vi "MarvinReport.vi"(0 "HEADER1":string="===================================================================\r\n||  Functional and Performance Test  For  DUAL-SERVO- L O W E R  ||\r\n||  P/N  TLM132XX501    S/N:001    Power-Input:18,28,32 +/-0.5V  ||\r\n||  Date:6/12/2007    Time: 15-00  Test-Conductor: Itzik         ||\r\n||  Tester P/N yyyy-yyyyyy-yyyy    S/N:01                        ||\r\n||  POWER SUPPLY P/N xxxxx                                       ||\r\n||  Remarks:                                                     ||\r\n||  You can write here what ever you want                        ||\r\n||                                                               ||\r\n===================================================================", 1 "ATR Or":refnum<vi>, 2 "Steps   pfull":string[][](table)=array602x15[9030 elements] caption="ATR", 5 "pageNum":i32=13, 7 "FILE NAME":string="d", 9 "Report Folder":path=path "C:/EPD/ATRS", 11 "Open File":bool caption="Open", 12 "error in (no error)":errorcluster, 14 "Test-Conductor":string) -> (4 "path out":path, 15 "error out":errorcluster)   [LabVIEW 2017]
uses:
  <vilib>/Utility/miscctls.llb/LVRowAndColumnUnsignedTypeDef.ctl
  <vilib>/Utility/NIReport.llb/Append Report Text (str wrap).vi
  <vilib>/Utility/NIReport.llb/NI_report.lvclass
  <vilib>/Utility/NIReport.llb/Word/NI_Word.lvclass
panel:
  out "error out 2":errorcluster
  out "RefArr":u32[](array[numeric])
  in  "Tab Control":T1(tab)=enum."Headers and more"
  out "ERRORS\nLIST":string="<pre>Summery of Results (Fails Only) :   Pos.Cmnd.=0.5V F.B. - FAIL !\t   \nPos.Cmnd.=2.0V F.B. - FAIL !\t       Pos.Cmnd.=4.5V F.B. - FAIL !\t  \nPos.Cmnd.=0.5V F.B  - FAIL !\t       Pos.Cmnd.=2.0V F.B. - FAIL !\t\nPos.Cmnd.=4.5V F.B. - FAIL !\t       Pot. / Pos.Cmnd. 1.5v - FAIL !\t   \nPot./Pos.Cmnd.2.0v  - FAIL !\t       Pot. / Pos.Cmnd. 3.5v - FAIL !\t   \nRelay-->RESET  - FAIL !\t            Relay --> SET - FAIL !\t</pre>"
  out "Steps   p1":string[][](table)=[["Load Firmware - reset", "-", "-", "-", "-", ""], ["Test Communication", "-", "-", "-", "-", ""], ["Set S/N", "-", "-", "-", "-", ""], ["Set Board Number", "-", "-", "-", "-", ""], [" ", "", "", "", "", ""], ["Test Communication", "-", "-", "-", "-", ""], ["Get S/N", "-", "-", "-", "", ""], ["Get Board Number", "-", "-", "-", "", ""], ["Get FW", "-", "-", "-", "", ""], ["Small position command", "", "", "", "", ""], ["Measure delta", "", "", "", "", ""], ["Velocity command", "", "", "", "", ""], ["Velocity command", "", "", "", "", ""], ["Velocity command", "", "", "", "", ""], ["Velocity command", "", "", "", "", ""], ["Velocity command", "", "", "", "", ""]] caption="ATR"
  out "Steps   p2":string[][](table)=[["Load Firmware - reset", "-", "-", "-", "-", ""], ["Test Communication", "-", "-", "-", "-", ""], ["Set S/N", "-", "-", "-", "-", ""], ["Set Board Number", "-", "-", "-", "-", ""], [" ", "", "", "", "", ""], ["Test Communication", "-", "-", "-", "-", ""], ["Get S/N", "-", "-", "-", "", ""], ["Get Board Number", "-", "-", "-", "", ""], ["Get FW", "-", "-", "-", "", ""], ["Small position command", "", "", "", "", ""], ["Measure delta", "", "", "", "", ""], ["Velocity command", "", "", "", "", ""], ["Velocity command", "", "", "", "", ""], ["Velocity command", "", "", "", "", ""], ["Velocity command", "", "", "", "", ""], ["Velocity command", "", "", "", "", ""]] caption="ATR"
  out "Steps   p3":string[][](table) caption="ATR"
  in  "Fail  Button":bool
  in  "Pass  Button":bool
  # "e"
  # "e"
  # "<pre>"
  # "for html"
  # "for html"
  # "</pre>"
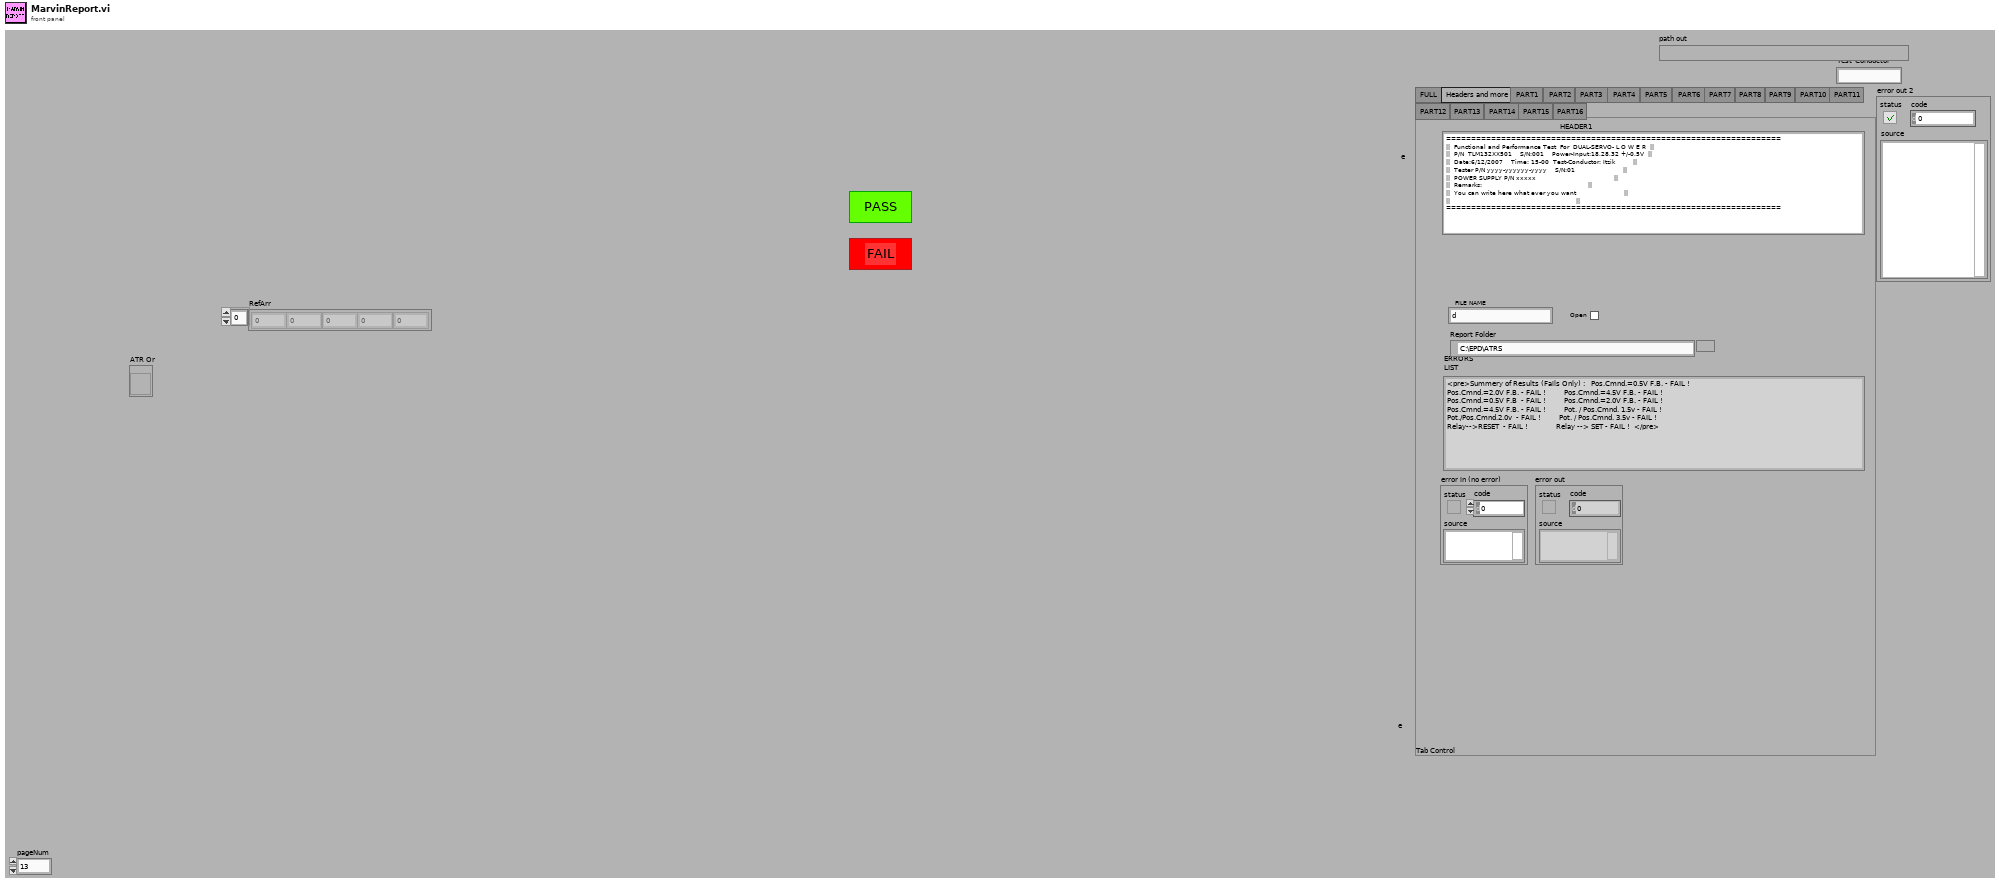
[diagram p1: front panel]
types:
  T1 = enum32{"FULL", "Headers and more", "PART1 ", "PART2 ", "PART3 ", "PART4 ", "PART5 ", "PART6 ", "PART7", "PART8", "PART9", "PART10", "PART11", "PART12", "PART13", "PART14", "PART15", "PART16"}
  T2 = typedef "LVRowAndColumnUnsignedTypeDef.ctl" = cluster{"Row":u32, "Column":u32}
  T3 = enum16{"Standard Report", "HTML", "Word", "Excel"}
  T4 = cluster{"Italic":enum16{"Italic Unchanged", "Italic On", "Italic Off"}, "Strike Through":enum16{"Strike Through Unchanged", "Strike Through On", "Strike Through Off"}, "Underline":enum16{"Underline Unchanged", "Underline On", "Underline Off"}, "Bold":enum16{"Bold Unchanged", "Bold On", "Bold Off"}}
  T5 = cluster{"charset (-1)":i16, "weight (-1)":i16, "name":string, "size":string}
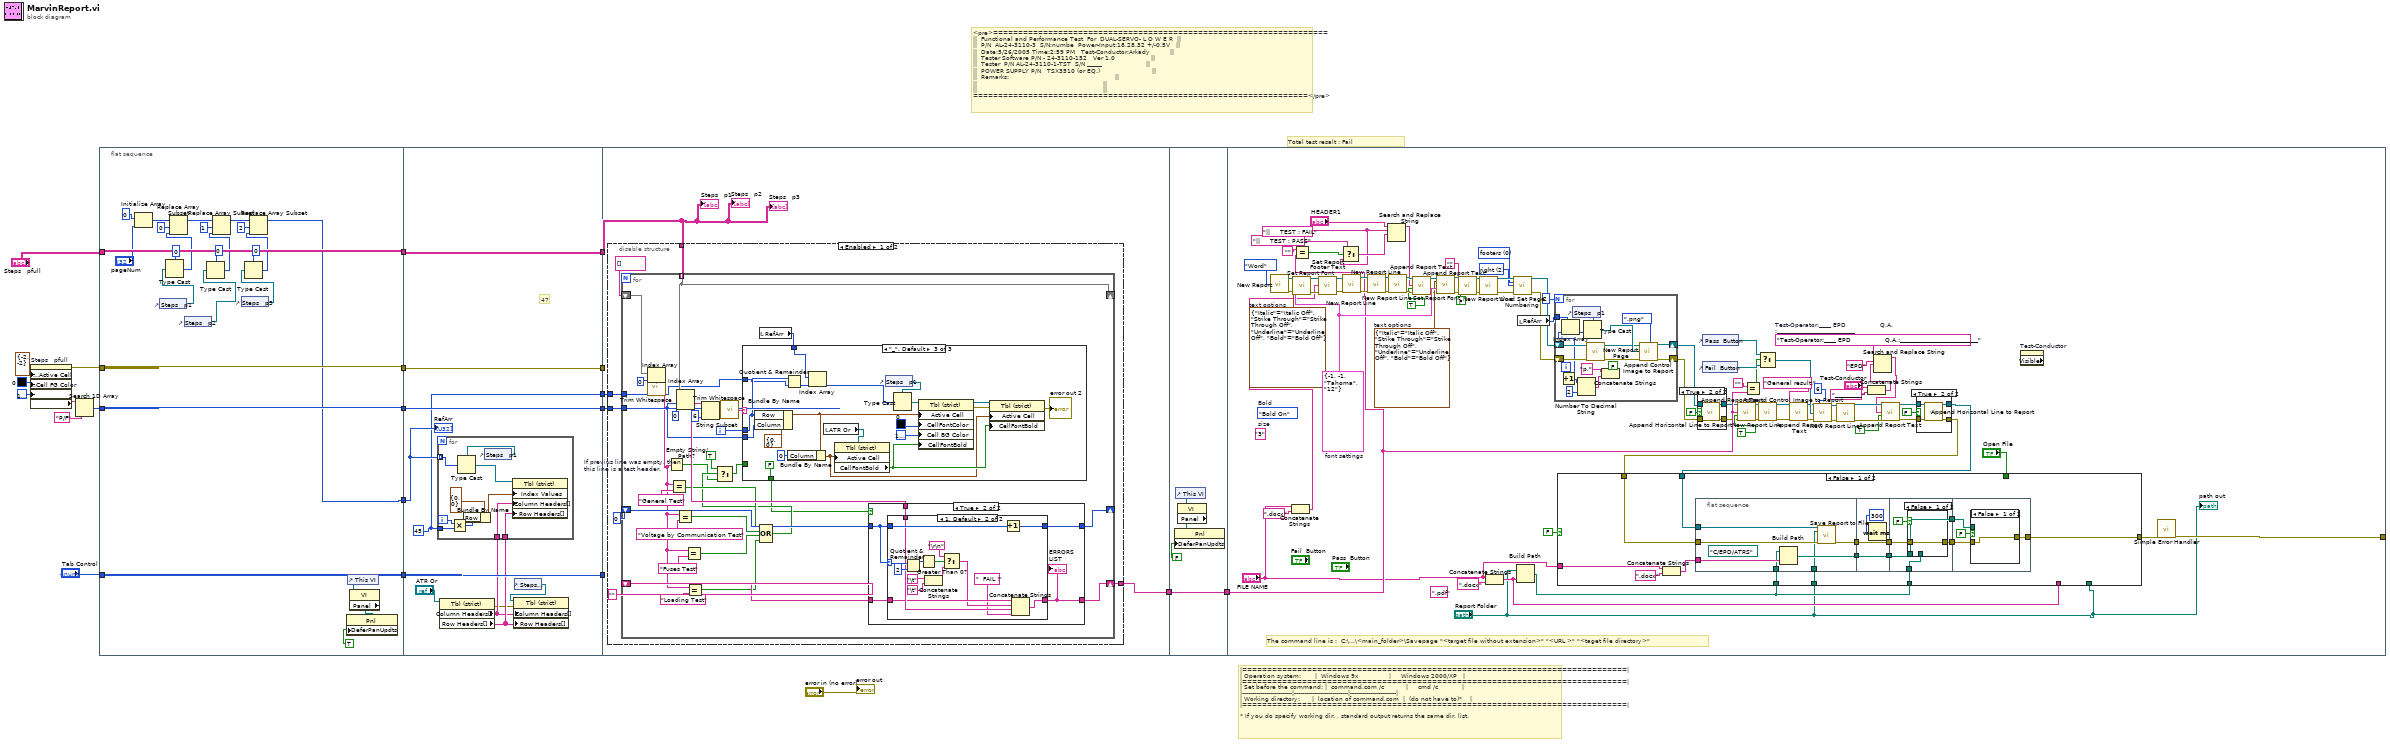
[diagram p0: block diagram]
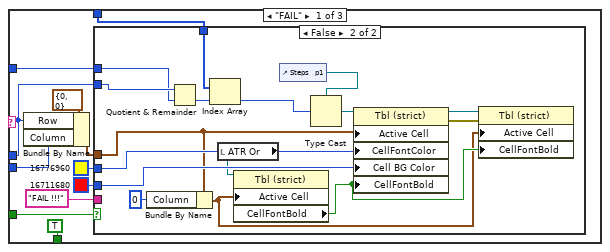
[diagram p2: hidden frame]
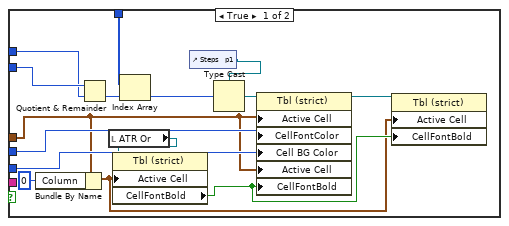
[diagram p3: hidden frame]
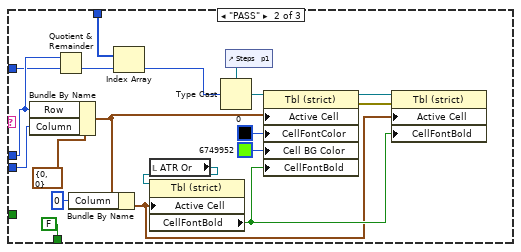
[diagram p4: hidden frame]
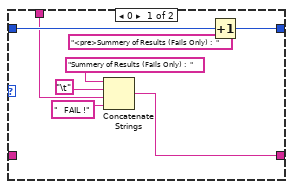
[diagram p6: hidden frame]
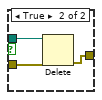
[diagram p9: hidden frame]
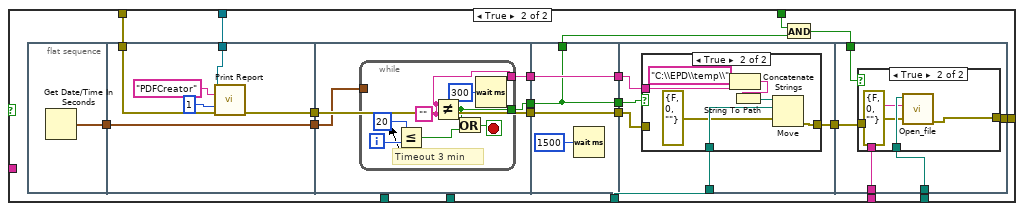
[diagram p10: hidden frame]
diagram:
  # "Total test resalt : Fail"
  # "|=============================================================================|\n| Operation system:       |  Windows 9x               |     Windows 2000/XP   |\n|=============================================================================|\n| Set before the command: |  command.com /c           |     cmd /c            |\n|-------------------------|---------------------------|-----------------------|\n| Working directory:      |  location of command.com  |  (do not have to)*    |\n|=============================================================================|\n\n* If you do specify working dir. , standard output returns the same dir. list."
  # "<pre>===================================================================\n||  Functional and Performance Test  For  DUAL-SERVO- L O W E R  ||\n||  P/N  AL-24-3110-3  S/N:numbe  Power-Input:18,28,32 +/-0.5V   ||\n||  Date:5/26/2005 Time:2:59 PM   Test-Conductor:Arkady          ||\n||  Tester Software P/N - 24-3110-152   Ver 1.0                  ||\n||  Tester  P/N AL-24-3110-1-TST  S/N _____                      ||\n||  POWER SUPPLY P/N   TSX3510 (or EQ.)                          ||\n||  Remarks:                                                     ||\n||                                                               ||\n||                                                               ||\n===================================================================</pre>"
  n1 = property on="Steps   pfull" class="Tbl (strict)"("Active Cell:Active Cell"=cluster{"Row":i32, "Column":i32} {"Row"=-2, "Column"=-2} ("Active Cell"), "Active Cell:Cell FG Color"=u32 0, "Active Cell:Cell Background Color"=u32 16777226) -> (error out=w19:errorcluster, "Column Header Strings[]"=w17:string[])  [unwired: 2 in, 1 out]
  n2 = Search 1D Array(1D array=w17, element="P/F") -> (index of element=w16:i32)  [unwired: 1 in]
  n3 = flat-sequence {
    tunnel: "Tab Control" -> [w44]
    tunnel: w16 -> [w45]
    tunnel: w19 -> [w46]
    tunnel: "Steps   pfull" -> [w47]
    tunnel: [w47] -> w8
    tunnel: [w46] -> w7
    tunnel: [w45] -> w6
    tunnel: [w44] -> w5
    tunnel: [w23] -> w2
    tunnel: [w58] -> w12
    tunnel: [w57] -> w11
    tunnel: [w56] -> w10
    tunnel: [w55] -> w9
    tunnel: w8 -> [w58]
    tunnel: w7 -> [w57]
    tunnel: w6 -> [w56]
    tunnel: w5 -> [w55]
    tunnel: w2 -> [w50]
    tunnel: [w48] -> w1
    tunnel: [w71] -> w4
    tunnel: w12 -> [w70]
    tunnel: w11 -> [_]
    tunnel: w10 -> [w72]
    tunnel: w9 -> [_]
    tunnel: w1 -> [w69]
    tunnel: w4 -> [w225]
    tunnel: [w225] -> w3
    tunnel: [w309] -> _
    tunnel: w3 -> [w271]
    frame #0 {
      n4 = Initialize Array "Initialize Array"(u32 0, "pageNum") -> (w28:u32[])
      n5 = control-ref of="Steps   p1"() -> (w40:refnum<vi>)
      n6 = Type Cast(type=u32 0, x=w40) -> (*(type *) &x=w29:u32)
      n7 = Replace Array Subset(array=w28, new element=w29, index=0) -> (w32:u32[])
      n8 = control-ref of="Steps   p2"() -> (w24:refnum<vi>)
      n9 = Type Cast(type=u32 0, x=w24) -> (*(type *) &x=w33:u32)
      n10 = Replace Array Subset(array=w32, new element=w33, index=1) -> (w38:u32[])
      n11 = control-ref of="Steps   p3"() -> (w39:refnum<vi>)
      n12 = Type Cast(type=u32 0, x=w39) -> (*(type *) &x=w36:u32)
      n13 = Replace Array Subset(array=w38, new element=w36, index=2) -> (w23:u32[])
      n14 = control-ref of="This VI"() -> (w41:refnum<vi>)
      n15 = property class="VI"(reference=w41) -> ("Panel"=w42:refnum<vi>)  [unwired: 1 in, 2 out]
      n16 = property class="Pnl"(reference=w42, "DeferPanUpdts"=TRUE ("Defer Panel Updates")) -> ()  [unwired: 1 in, 2 out]
    }
    frame #1 {
      w48 = u32 45 ("Row")
      # "47"
      n17 = property class="Tbl (strict)"(reference="ATR Or") -> (error out=w52:errorcluster, "Column Headers[]"=w53:string[], "Row Headers[]"=w54:string[])  [unwired: 1 in, 1 out]
      n18 = for {
        tunnel: w50 -> [w68] mode=indexing
        tunnel: w53 -> [w62]
        tunnel: w54 -> [w61]
        tunnel: w48 -> [w59]
        i -> [w64]
        n19 = Multiply(x=w64, y=w59) -> (x*y=w63:u32)
        n20 = Bundle By Name(cluster=T2 {"Row"=0, "Column"=0} ("Index Values"), "Row"=w63) -> (w65:T2)
        n21 = control-ref of="Steps   p1"() -> (w60:refnum<vi>)
        n22 = Type Cast(type=w60, x=w68) -> (*(type *) &x=w67:refnum<vi>)
        n23 = property class="Tbl (strict)"(reference=w67, "Index Values"=w65, "Column Headers[]"=w62, "Row Headers[]"=w61) -> ()  [unwired: 1 in, 2 out]
      }
      n24 = control-ref of="Steps   pfull"() -> (w49:refnum<vi>)
      n25 = property class="Tbl (strict)"(reference=w49, error in=w52, "Column Headers[]"=w53, "Row Headers[]"=w54) -> ()  [unwired: 2 out]
      "RefArr" <- w50
    }
    frame #2 {
      n26 = disable-structure shown="Enabled" {
        disable-tunnel: w72 -> [w79 _]
        disable-tunnel: [w78 _] -> w71
        disable-tunnel: w70 -> [w74 _]
        disable-tunnel: w69 -> [w73 _]
        frame Enabled {
          n27 = for {
            tunnel: w74 -> [w109] mode=indexing
            shift-right: [w109] -> _
            shift-left: string[] [] ("ATR in") -> [w108]
            tunnel: w79 -> [w85]
            shift-right: [w100] -> w78
            shift-left: "" ("trimmed string") -> [w104]
            shift-right: [w103] -> _
            shift-left: 0 -> [w102]
            tunnel: w73 -> [w80]
            i -> [w86]
            n28 = Index Array(array=w108, index=0) -> (element=w106:string)
            n29 = call <vilib>:"Trim Whitespace.vi"("string"=w106) -> ("trimmed string"=w81:string)  [unwired: 1 in]
            n30 = Empty String/Path? "If previus line was empty, then\nthis line is a test header."(string/path=w81) -> (empty?=w88:bool)
            n31 = Equal?(x=w81, y="General Test") -> (x = y?=w97:bool)
            n32 = Equal?(x=w81, y="Voltage by Communication Test") -> (x = y?=w92:bool)
            n33 = Index Array(array=w109, index #1=w85, index #2=0) -> (element #1=w105:string, element #2=w101:string)
            n34 = Equal?(x=w81, y="Fuses Test") -> (x = y?=w93:bool)
            n35 = Equal?(x=w81, y="Loading Test") -> (x = y?=w94:bool)
            n36 = String Subset(string=w105, length (rest)=6 ("length (rest)")) -> (substring=w110:string)  [unwired: 1 in]
            n37 = call <vilib>:"Trim Whitespace.vi"("string"=w110) -> ("trimmed string"=w87:string)  [unwired: 1 in]
            n38 = local read "RefArr"() -> (w82:u32[])
            n39 = Compound Arithmetic op=OR(w97, w92, w93, w94) -> (w95:bool)
            n40 = Select(t=TRUE, s=w95, f=w88) -> (s? t:f=w84:bool)
            n41 = case shown="\"_\", Default" w87 {
              tunnel: w86 -> [w114 w167 w188]
              tunnel: w85 -> [w116 w171 w191]
              tunnel: w84 -> [w118 _ _]
              tunnel: [TRUE FALSE FALSE] -> w83
              tunnel: w82 -> [w115 w165 w187]
              tunnel: w80 -> [w112 w154 w173]
              frame "FAIL" {
                n42 = Bundle By Name(cluster=cluster{"Row":i32, "Column":i32} {"Row"=0, "Column"=0} ("Active Cell"), "Row"=w114, "Column"=w116) -> (w122:cluster{"Row":i32, "Column":i32})
                n43 = case shown="False" w118 {
                  tunnel: w122 -> [w130 w142]
                  tunnel: u32 16776960 -> [w137 w153]
                  tunnel: u32 16711680 -> [w136 w152]
                  tunnel: "FAIL !!!" ("string") -> [_ _]
                  tunnel: w115 -> [w134 w149]
                  tunnel: w114 -> [w133 w150]
                  tunnel: w112 -> [w123 w138]
                  frame True {
                    n44 = Bundle By Name(cluster=w130, "Column"=0) -> (w126:cluster{"Row":i32, "Column":i32})
                    n45 = Quotient & Remainder(x=w133, y=w123) -> (floor(x/y)=w135:u32)  [unwired: 1 out]
                    n46 = local read "ATR Or"() -> (w124:refnum<vi>)
                    n47 = property class="Tbl (strict)"(reference=w124, "Active Cell"=w126) -> ("CellFontBold"=w127:bool)  [unwired: 1 in, 2 out]
                    n48 = Index Array(array=w134, index=w135) -> (element=w131:u32)
                    n49 = control-ref of="Steps   p1"() -> (w125:refnum<vi>)
                    n50 = Type Cast(type=w125, x=w131) -> (*(type *) &x=w132:refnum<vi>)
                    n51 = property class="Tbl (strict)"(reference=w132, "Active Cell"=w130, "CellFontColor"=w137, "Cell BG Color"=w136, "Active Cell"=w130, "CellFontBold"=w127) -> (reference out=w128:refnum<vi>)  [unwired: 1 in, 1 out]
                    n52 = property class="Tbl (strict)"(reference=w128, "Active Cell"=w126, "CellFontBold"=w127) -> ()  [unwired: 1 in, 2 out]
                  }
                  frame False {
                    n53 = Bundle By Name(cluster=w142, "Column"=0) -> (w141:cluster{"Row":i32, "Column":i32})
                    n54 = Quotient & Remainder(x=w150, y=w138) -> (floor(x/y)=w151:u32)  [unwired: 1 out]
                    n55 = Index Array(array=w149, index=w151) -> (element=w148:u32)
                    n56 = local read "ATR Or"() -> (w140:refnum<vi>)
                    n57 = property class="Tbl (strict)"(reference=w140, "Active Cell"=w141) -> ("CellFontBold"=w144:bool)  [unwired: 1 in, 2 out]
                    n58 = control-ref of="Steps   p1"() -> (w139:refnum<vi>)
                    n59 = Type Cast(type=w139, x=w148) -> (*(type *) &x=w147:refnum<vi>)
                    n60 = property class="Tbl (strict)"(reference=w147, "Active Cell"=w142, "CellFontColor"=w153, "Cell BG Color"=w152, "CellFontBold"=w144) -> (reference out=w146:refnum<vi>, error out=w145:errorcluster)  [unwired: 1 in]
                    n61 = property class="Tbl (strict)"(reference=w146, error in=w145, "Active Cell"=w141, "CellFontBold"=w144) -> ()  [unwired: 2 out]
                  }
                }
              }
              frame "PASS" {
                n62 = Bundle By Name(cluster=cluster{"Row":i32, "Column":i32} {"Row"=0, "Column"=0} ("Active Cell"), "Row"=w167, "Column"=w171) -> (w158:cluster{"Row":i32, "Column":i32})
                n63 = Quotient & Remainder(x=w167, y=w154) -> (floor(x/y)=w166:u32)  [unwired: 1 out]
                n64 = Bundle By Name(cluster=w158, "Column"=0) -> (w157:cluster{"Row":i32, "Column":i32})
                n65 = Index Array(array=w165, index=w166) -> (element=w164:u32)
                n66 = local read "ATR Or"() -> (w155:refnum<vi>)
                n67 = property class="Tbl (strict)"(reference=w155, "Active Cell"=w157) -> ("CellFontBold"=w160:bool)  [unwired: 1 in, 2 out]
                n68 = control-ref of="Steps   p1"() -> (w156:refnum<vi>)
                n69 = Type Cast(type=w156, x=w164) -> (*(type *) &x=w163:refnum<vi>)
                n70 = property class="Tbl (strict)"(reference=w163, "Active Cell"=w158, "CellFontColor"=u32 0, "Cell BG Color"=u32 6749952, "CellFontBold"=w160) -> (reference out=w161:refnum<vi>, error out=w162:errorcluster)  [unwired: 1 in]
                n71 = property class="Tbl (strict)"(reference=w161, error in=w162, "Active Cell"=w157, "CellFontBold"=w160) -> ()  [unwired: 2 out]
              }
              frame "_", Default {
                n72 = Bundle By Name(cluster=cluster{"Row":i32, "Column":i32} {"Row"=0, "Column"=0} ("Active Cell"), "Row"=w188, "Column"=w191) -> (w181:cluster{"Row":i32, "Column":i32})
                n73 = Quotient & Remainder(x=w188, y=w173) -> (floor(x/y)=w189:u32)  [unwired: 1 out]
                n74 = Bundle By Name(cluster=w181, "Column"=0) -> (w177:cluster{"Row":i32, "Column":i32})
                n75 = Index Array(array=w187, index=w189) -> (element=w186:u32)
                n76 = local read "ATR Or"() -> (w175:refnum<vi>)
                n77 = property class="Tbl (strict)"(reference=w175, "Active Cell"=w177) -> ("CellFontBold"=w178:bool)  [unwired: 1 in, 2 out]
                n78 = control-ref of="Steps   p1"() -> (w176:refnum<vi>)
                n79 = Type Cast(type=w176, x=w186) -> (*(type *) &x=w183:refnum<vi>)
                n80 = property class="Tbl (strict)"(reference=w183, "Active Cell"=w181, "CellFontColor"=u32 0, "Cell BG Color"=u32 16777226, "CellFontBold"=w178) -> (reference out=w180:refnum<vi>, error out=w179:errorcluster)  [unwired: 1 in]
                n81 = property class="Tbl (strict)"(reference=w180, error in=w179, "Active Cell"=w177, "CellFontBold"=w178) -> (error out=→"error out 2":errorcluster)  [unwired: 1 out]
              }
            }
            n82 = case shown="True" w83 {
              tunnel: w104 -> [w194 w196]
              tunnel: [w194 w195] -> w100
              tunnel: w102 -> [w193 w198]
              tunnel: [w193 w199] -> w103
              tunnel: w101 -> [_ w197]
              frame False {
              }
              frame True {
                n83 = case shown="1, Default" w198 {
                  selector: w198 -> [_ w220]
                  tunnel: [w201 w210] -> w199
                  tunnel: w198 -> [w206 w221]
                  tunnel: w197 -> [w205 w217]
                  tunnel: [w203 w216] -> w195
                  tunnel: w196 -> [_ w215]
                  frame 0 {
                    (unwired) "<pre>Summery of Results (Fails Only) :  "
                    n84 = Concatenate Strings("Summery of Results (Fails Only) :  ", "\t", w205, "  FAIL !" ("string")) -> (w203:string)
                    n85 = Increment(x=w206) -> (x+1=w201:i32)
                  }
                  frame 1, Default {
                    n86 = Quotient & Remainder(x=w220, y=2) -> (x-y*floor(x/y)=w218:i32)  [unwired: 1 out]
                    n87 = Greater Than 0?(x=w218) -> (x > 0?=w214:bool)
                    n88 = Concatenate Strings("\t", "\t") -> (w209:string)
                    n89 = Select(t="\r\n", s=w214, f=w209) -> (s? t:f=w212:string)
                    n90 = Increment(x=w221) -> (x+1=w210:i32)
                    n91 = Concatenate Strings(w215, w212, w217, "  FAIL !" ("string")) -> (w216:string)
                  }
                }
                "ERRORS\nLIST" <- w195
              }
            }
          }
        }
        frame Disabled {
        }
      }
      "Steps   p1" <- w70
      "Steps   p3" <- w70
      "Steps   p2" <- w70
    }
    frame #3 {
      n92 = control-ref of="This VI"() -> (w222:refnum<vi>)
      n93 = property class="VI"(reference=w222) -> ("Panel"=w223:refnum<vi>)  [unwired: 1 in, 2 out]
      n94 = property class="Pnl"(reference=w223, "DeferPanUpdts"=FALSE ("Defer Panel Updates")) -> ()  [unwired: 1 in, 2 out]
    }
    frame #4 {
      w231 = u16 2 items=["left", "center", "right"] ("alignment (right)")
      w232 = u16 0 items=["footers", "headers"] ("position (footers)")
      (unwired) ".pdf" ("File Name")
      (unwired) "3"  # size
      (unwired) enum16{"Bold Unchanged", "Bold On", "Bold Off"}."Bold On"  # Bold
      w272 = "||     TEST : FAIL"
      w278 = T4 {"Italic"=enum."Italic Off", "Strike Through"=enum."Strike Through Off", "Underline"=enum."Underline Off", "Bold"=enum."Bold Off"}  # text options
      w312 = T4 {"Italic"=enum."Italic Off", "Strike Through"=enum."Strike Through Off", "Underline"=enum."Underline Off", "Bold"=enum."Bold Off"}  # text options
      w267 = "Test-Operator:____ EPD                 Q.A.:__________________________"  # Test-Operator:____ EPD                 Q.A.:__________________________
      w279 = T5 {"charset (-1)"=-1, "weight (-1)"=-1, "name"="Tahoma", "size"="12"}  # font settings
      # "The command line is :  C:\\...\\<main_folder>\\Savepage \"<target file without extension>\" \"<URL >\" \"<taget file directory>\""
      n95 = call <vilib>:"New Report.vi"("report type"=T3."Word") -> ("report out"=w310:refnum<class "NI_report.lvclass">, "error out"=w311:errorcluster)  [unwired: 13 in]
      n96 = Concatenate Strings("FILE NAME", ".docx" ("File Name")) -> (w250:string)
      n97 = call-dynamic "Set Report Font.vi"("report in"=w310, "text options"=w312, "font settings"=w279, "error in (no error)"=w311) -> ("report out"=w255:refnum<class "NI_report.lvclass">, "error out"=w252:errorcluster)  [unwired: 9 in, 1 out]
      n98 = Equal?(x="", y=w271) -> (x = y?=w274:bool)
      n99 = call-dynamic "Set Report Footer Text.vi"("report in"=w255, "center footer text"=w250, "error in (no error)"=w252) -> ("report out"=w254:refnum<class "NI_report.lvclass">, "error out"=w253:errorcluster)  [unwired: 11 in]
      n100 = Select(t="||     TEST : PASS", s=w274, f=w272) -> (s? t:f=w276:string)
      n101 = call-dynamic "New Report Line.vi"("report in"=w254, "error in (no error)"=w253) -> ("report out"=w281:refnum<class "NI_report.lvclass">, "error out"=w280:errorcluster)  [unwired: 12 in]
      n102 = call-dynamic "New Report Line.vi"("report in"=w281, "error in (no error)"=w280) -> ("report out"=w284:refnum<class "NI_report.lvclass">, "error out"=w285:errorcluster)  [unwired: 12 in]
      n103 = Search and Replace String(input string="HEADER1", search string=w272, replace string=w276) -> (result string=w259:string)  [unwired: 5 in, 3 out]
      n104 = call-dynamic "New Report Line.vi"("report in"=w284, "error in (no error)"=w285) -> ("report out"=w288:refnum<class "NI_report.lvclass">, "error out"=w287:errorcluster)  [unwired: 12 in]
      n105 = call-poly <vilib>:"Append Report Text.vi"("report in"=w288, "text"=w259, "append on new line? (F)"=TRUE, "error in (no error)"=w287) -> ("report out"=w261:refnum<class "NI_report.lvclass">, "error out"=w260:errorcluster)  [unwired: 8 in, 2 out]
      n106 = call-dynamic "Set Report Font.vi"("report in"=w261, "text options"=w278, "font settings"=w279, "error in (no error)"=w260) -> ("report out"=w282:refnum<class "NI_report.lvclass">, "error out"=w283:errorcluster)  [unwired: 9 in, 1 out]
      n107 = call-poly <vilib>:"Append Report Text.vi"("report in"=w282, "text"="", "append on new line? (F)"=FALSE, "error in (no error)"=w283) -> ("report out"=w306:refnum<class "NI_report.lvclass">, "error out"=w307:errorcluster)  [unwired: 8 in, 2 out]
      n108 = call-dynamic "New Report Line.vi"("report in"=w306, "error in (no error)"=w307) -> ("report out"=w236:refnum<class "NI_report.lvclass">, "error out"=w235:errorcluster)  [unwired: 12 in]
      n109 = Concatenate Strings("FILE NAME", ".docx" ("File Name")) -> (w239:string)
      n110 = call <vilib>:"Word Set Page Numbering.vi"("report in"=w236, "position (footers)"=w232, "alignment (right)"=w231, "error in (no error)"=w235) -> ("report out"=w234:refnum<class "NI_report.lvclass">, "error out"=w233:errorcluster)  [unwired: 10 in]
      n111 = Build Path(base path="Report Folder", name or relative path=w239) -> (appended path=w228:path)
      n112 = local read "RefArr"() -> (w229:u32[])
      n113 = for {
        N: 2 -> [_]
        tunnel: w229 -> [w419]
        shift-right: [w426] -> w245
        shift-left: w233 -> [w427]
        shift-right: [w425] -> w244
        shift-left: w234 -> [w428]
        i -> [w417]
        (unwired) FALSE ("append on new line? (F)")
        n114 = Increment(x=w417) -> (x+1=w431:i32)
        n115 = Index Array(array=w419, index=w417) -> (element=w418:u32)
        n116 = control-ref of="Steps   p1"() -> (w423:refnum<vi>)
        n117 = Number To Decimal String(number=w431, width (-)=i16 2) -> (decimal integer string=w429:string)
        n118 = Type Cast(type=w423, x=w418) -> (*(type *) &x=w424:refnum<vi>)
        n119 = call-dynamic "New Report Page.vi"("report in"=w428, "error in (no error)"=w427) -> ("report out"=w421:refnum<class "NI_report.lvclass">, "error out"=w420:errorcluster)  [unwired: 12 in]
        n120 = Concatenate Strings("p.", w429) -> ()  [unwired: 1 out]
        n121 = call-dynamic "Append Control Image to Report.vi"("report in"=w421, "image file type (.jpg)"=enum16{".jpg", ".png"}.".png" ("image file type(.jpg)"), "ctrl reference"=w424, "error in (no error)"=w420) -> ("report out"=w425:refnum<class "NI_report.lvclass">, "error out"=w426:errorcluster)  [unwired: 8 in, 2 out]
      }
      n122 = case shown="True" FALSE {
        tunnel: [w433 w438] -> w270
        tunnel: [w434 w437] -> w269
        tunnel: w245 -> [w433 w436]
        tunnel: w244 -> [w434 w435]
        frame False {
        }
        frame True {
          n123 = call-dynamic "Append Horizontal Line to Report.vi"("report in"=w435, "error in (no error)"=w436) -> ("report out"=w437:refnum<class "NI_report.lvclass">, "error out"=w438:errorcluster)  [unwired: 12 in]
        }
      }
      n124 = control-ref of="Fail  Button"() -> (w299:refnum<vi>)
      n125 = control-ref of="Pass  Button"() -> (w300:refnum<vi>)
      n126 = call-poly <vilib>:"Append Report Text.vi"("report in"=w269, "text"=w271, "append on new line? (F)"=TRUE, "error in (no error)"=w270) -> ("report out"=w304:refnum<class "NI_report.lvclass">, "error out"=w303:errorcluster)  [unwired: 8 in, 2 out]
      n127 = Equal?(x="", y=w271) -> (x = y?=w297:bool)
      n128 = Select(t=w300, s=w297, f=w299) -> (s? t:f=w301:refnum<vi>)
      n129 = call-dynamic "New Report Line.vi"("report in"=w304, "error in (no error)"=w303) -> ("report out"=w289:refnum<class "NI_report.lvclass">, "error out"=w290:errorcluster)  [unwired: 12 in]
      n130 = call-poly <vilib>:"Append Report Text.vi"("report in"=w289, "text"="General result:", "error in (no error)"=w290) -> ("report out"=w295:refnum<class "NI_report.lvclass">, "error out"=w296:errorcluster)  [unwired: 9 in, 2 out]
      n131 = call-dynamic "Append Control Image to Report.vi"("report in"=w295, "alignment (default)"=6, "ctrl reference"=w301, "error in (no error)"=w296) -> ("report out"=w294:refnum<class "NI_report.lvclass">, "error out"=w293:errorcluster)  [unwired: 8 in, 2 out]
      n132 = call-dynamic "New Report Line.vi"("report in"=w294, "error in (no error)"=w293) -> ("report out"=w291:refnum<class "NI_report.lvclass">, "error out"=w292:errorcluster)  [unwired: 12 in]
      n133 = Concatenate Strings("Test-Conductor", "_________") -> (w262:string)
      n134 = Search and Replace String(input string=w267, search string="EPD", replace string=w262) -> (result string=w264:string)  [unwired: 5 in, 3 out]
      n135 = call-poly <vilib>:"Append Report Text.vi"("report in"=w291, "text"=w264, "append on new line? (F)"=TRUE, "error in (no error)"=w292) -> ("report out"=w257:refnum<class "NI_report.lvclass">, "error out"=w256:errorcluster)  [unwired: 8 in, 2 out]
      n136 = case shown="True" FALSE {
        tunnel: w257 -> [w440 w444]
        tunnel: w256 -> [w439 w443]
        tunnel: [w439 w442] -> w243
        tunnel: [w440 w441] -> w241
        frame False {
        }
        frame True {
          n137 = call-dynamic "Append Horizontal Line to Report.vi"("report in"=w444, "error in (no error)"=w443) -> ("report out"=w441:refnum<class "NI_report.lvclass">, "error out"=w442:errorcluster)  [unwired: 12 in]
        }
      }
      n138 = case shown="False" FALSE {
        tunnel: [w323 w361] -> w238
        tunnel: w243 -> [w327 w360]
        tunnel: w228 -> [w319 w359]
        tunnel: w239 -> [_ w358]
        tunnel: "Report Folder" -> [_ w357]
        tunnel: w241 -> [w326 w356]
        tunnel: "Open File" -> [_ w354]
        tunnel: "FILE NAME" -> [w317 _]
        tunnel: w228 -> [w314 _]
        tunnel: "Report Folder" -> [w313 _]
        frame False {
          n139 = Concatenate Strings(w317, ".docx" ("File Name")) -> (w315:string)
          n140 = flat-sequence {
            tunnel: w327 -> [w334]
            tunnel: w326 -> [w332]
            tunnel: [w333] -> w325
            tunnel: [w331] -> w322
            tunnel: w315 -> [w330]
            tunnel: w314 -> [w329]
            tunnel: w313 -> [w328]
            tunnel: w325 -> [w337]
            tunnel: [w337] -> w324
            tunnel: w322 -> [w335]
            tunnel: [w335] -> w321
            tunnel: w324 -> [w342]
            tunnel: w321 -> [w340]
            tunnel: [w338] -> w320
            tunnel: w319 -> [w341]
            tunnel: [w340] -> w318
            tunnel: [w347] -> w323
            tunnel: w320 -> [w348]
            tunnel: w318 -> [w346]
            frame #0 {
              (unwired) path "C:/EPD/ATRS" ("report file path")
              n141 = Build Path(base path=w329, name or relative path=w330) -> (appended path=w331:path)
              n142 = call-dynamic "Save Report to File.vi"("report in"=w332, "report file path"=w328, "error in (no error)"=w334) -> ("error out"=w333:errorcluster)  [unwired: 11 in, 1 out]
            }
            frame #1 {
              n143 = Wait (ms)(milliseconds to wait=u32 300) -> ()  [unwired: 1 out]
            }
            frame #2 {
              n144 = case shown="False" FALSE {
                tunnel: w342 -> [w343 w344]
                tunnel: w341 -> [_ _]
                tunnel: w340 -> [_ _]
                tunnel: [w343 w344] -> w338
                frame False {
                }
                frame True {
                }
              }
            }
            frame #3 {
              n145 = case shown="False" FALSE {
                tunnel: w348 -> [w349 w352]
                tunnel: [w349 w351] -> w347
                tunnel: w346 -> [_ w350]
                frame False {
                }
                frame True {
                  n146 = Delete(path (use dialog)=w350, error in=w352) -> (error out=w351:errorcluster)  [unwired: 3 in, 2 out]
                }
              }
            }
          }
        }
        frame True {
          n147 = flat-sequence {
            tunnel: [w372] -> w371
            tunnel: w356 -> [w376]
            tunnel: w360 -> [w375]
            tunnel: [w374] -> w370
            tunnel: [w373] -> w369
            tunnel: w371 -> [w373]
            tunnel: w370 -> [w382]
            tunnel: w369 -> [w381]
            tunnel: [w382] -> w368
            tunnel: [w380] -> w367
            tunnel: [w379] -> w366
            tunnel: w368 -> [w393]
            tunnel: w367 -> [w392]
            tunnel: w366 -> [w390]
            tunnel: [w393] -> w365
            tunnel: [w392] -> w364
            tunnel: [w390] -> w353
            tunnel: [w390] -> w363
            tunnel: w365 -> [w398]
            tunnel: w364 -> [w397]
            tunnel: w363 -> [w396]
            tunnel: w359 -> [w395]
            tunnel: [w394] -> w362
            tunnel: w362 -> [w411]
            tunnel: w357 -> [w410]
            tunnel: w358 -> [w409]
            tunnel: [w408] -> w361
            tunnel: w355 -> [w407]
            frame #0 {
              n148 = Get Date/Time In Seconds() -> (seconds since 1Jan1904=w372:timestamp)
            }
            frame #1 {
              n149 = call-dynamic "Print Report.vi"("report in"=w376, "printer name (default)"="PDFCreator", "number of copies (1)"=1, "error in (no error)"=w375) -> ("error out"=w374:errorcluster)  [unwired: 10 in, 1 out]
            }
            frame #2 {
              n150 = while {
                tunnel: w381 -> [_]
                tunnel: [w383] -> w380
                tunnel: [w384] -> w379
                i -> [w387]
                stop <- w388 stop-if-true
                w383 = ""
                # "Timeout 3 min"
                n151 = Less Or Equal?(x=20, y=w387) -> (x <= y?=w385:bool)
                n152 = Not Equal?(x=w383, y=w383) -> (x != y?=w384:bool)
                n153 = Or(x=w384, y=w385) -> (x .or. y?=w388:bool)
                n154 = Wait (ms)(milliseconds to wait=u32 300) -> ()  [unwired: 1 out]
              }
            }
            frame #3 {
              n155 = Wait (ms)(milliseconds to wait=u32 1500) -> ()  [unwired: 1 out]
            }
            frame #4 {
              n156 = case shown="True" w396 {
                tunnel: w398 -> [w399 _]
                tunnel: [w399 w406] -> w394
                tunnel: w397 -> [_ w404]
                tunnel: w395 -> [_ w401]
                frame False {
                }
                frame True {
                  n157 = Concatenate Strings("C:\\EPD\\temp\\", w404) -> (w403:string)
                  n158 = String To Path(string=w403) -> (path=w402:path)
                  n159 = Move(source path=w402, error in=errorcluster {"status"=FALSE, "code"=0, "source"=""}, 10:w401) -> (error out=w406:errorcluster)  [unwired: 2 in, 2 out]
                }
              }
            }
            frame #5 {
              n160 = case shown="True" w407 {
                tunnel: w411 -> [w412 _]
                tunnel: [w412 w416] -> w408
                tunnel: w410 -> [_ w415]
                tunnel: w409 -> [_ w414]
                frame False {
                }
                frame True {
                  n161 = call "Open_file.vi"("error in"=errorcluster {"status"=FALSE, "code"=0, "source"=""}, "File Name input"=w414, "Work-Place path\n(with the webarch.exe)"=w415) -> ("error out"=w416:errorcluster)  [unwired: 6 in]
                }
              }
            }
          }
          n162 = And(x=w354, y=w353) -> (x .and. y?=w355:bool)
        }
      }
      n163 = property on="Test-Conductor" class="Str" props=["Visible"]() -> ()  [unwired: 2 in, 3 out]
      n164 = call <vilib>:"Simple Error Handler.vi"("error in (no error)"=w238) -> ("error out"=w309:errorcluster)  [unwired: 4 in, 4 out]
      "path out" <- "Report Folder"
    }
  }
  "error out" <- "error in (no error)"
